vi "WriteHiSpeedDevice.vi"(4 "High Output Pins":T1, 5 "Data Control":T3, 6 "Wait Data Write":T2, 7 "Init Condition":T4 {"Chip Select Pin" items=["ADBUS3 Chip Select", "ADBUS4 GPIOL1", "ADBUS5 GPIOL2", "ADBUS6 GPIOL3", "ADBUS7 GPIOL4"]}, 8 "error in (no error)":errorcluster, 9 "Data Buffer":u8[](array[numeric]), 10 "Control Buffer":u8[](array[numeric]), 11 "Handle":u32) -> (0 "error out":errorcluster, 3 "Result":u32)   [LabVIEW 2010]
uses:
  FTCSPI.dll
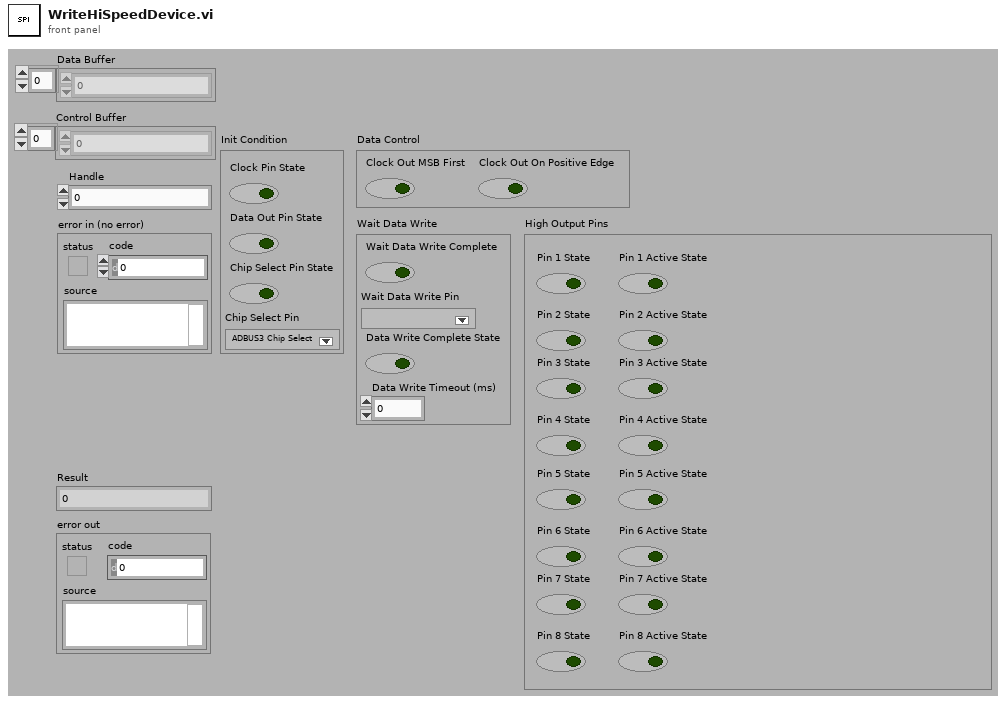
[diagram p1: front panel]
types:
  T1 = cluster{"Pin 1 State":bool, "Pin 1 Active State":bool, "Pin 2 State":bool, "Pin 2 Active State":bool, "Pin 3 State":bool, "Pin 3 Active State":bool, "Pin 4 State":bool, "Pin 4 Active State":bool, "Pin 5 State":bool, "Pin 5 Active State":bool, "Pin 6 State":bool, "Pin 6 Active State":bool, "Pin 7 State":bool, "Pin 7 Active State":bool, "Pin 8 State":bool, "Pin 8 Active State":bool}
  T2 = cluster{"Wait Data Write Complete":bool, "Wait Data Write Pin":u16, "Data Write Complete State":bool, "Data Write Timeout (ms)":u32}
  T3 = cluster{"Clock Out MSB First":bool, "Clock Out On Positive Edge":bool}
  T4 = cluster{"Clock Pin State":bool, "Data Out Pin State":bool, "Chip Select Pin State":bool, "Chip Select Pin":u16}
  T5 = cluster{u32, "Wait Data Write Pin":u16, u32, "Data Write Timeout (ms)":u32}
  T6 = cluster{"[0]":u32, "[1]":u32, "[2]":u32, "[3]":u32, "[4]":u32, "[5]":u32, "[6]":u32, "[7]":u32, "[8]":u32}
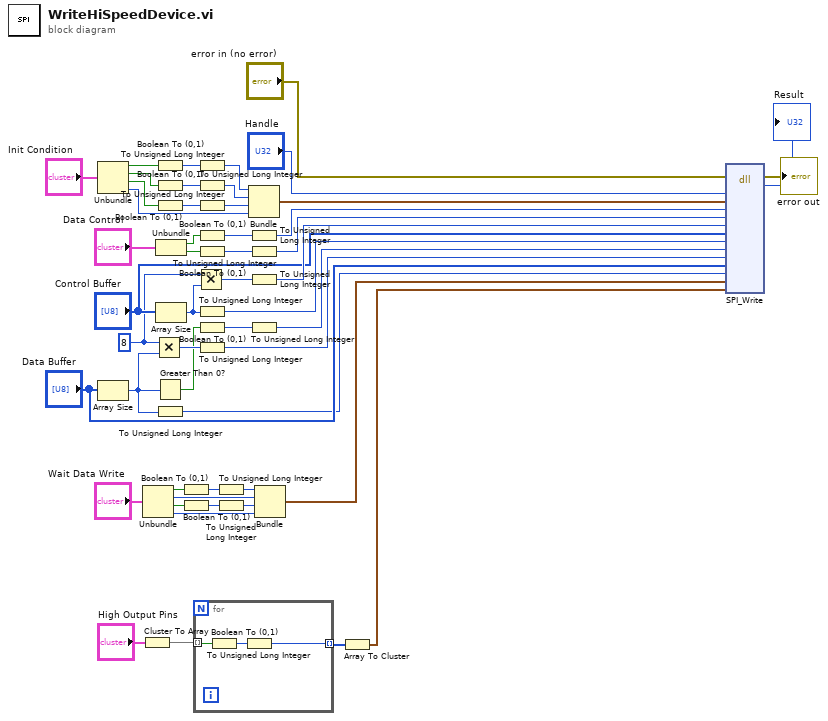
[diagram p0: block diagram]
diagram:
  w23 = 8
  n1 = Unbundle("Init Condition") -> ("Clock Pin State"=w48:bool, "Data Out Pin State"=w47:bool, "Chip Select Pin State"=w46:bool, "Chip Select Pin"=w42:u16)
  n2 = Array Size(array="Data Buffer") -> (size(s)=w17:i32)
  n3 = Cluster To Array(cluster="High Output Pins") -> (array=w5:bool[])
  n4 = Unbundle("Wait Data Write") -> ("Wait Data Write Complete"=w15:bool, "Wait Data Write Pin"=w9:u16, "Data Write Complete State"=w14:bool, "Data Write Timeout (ms)"=w8:u32)
  n5 = Multiply(x=w23, y=w17) -> (x*y=w24:i32)
  n6 = Boolean To (0,1)(Boolean=w48) -> (0, 1=w45:i16)
  n7 = Boolean To (0,1)(Boolean=w47) -> (0, 1=w43:i16)
  n8 = Boolean To (0,1)(Boolean=w46) -> (0, 1=w44:i16)
  n9 = Greater Than 0?(x=w17) -> (x > 0?=w21:bool)
  n10 = To Unsigned Long Integer(number=w17) -> (unsigned 32bit integer=w18:u32)
  n11 = Unbundle("Data Control") -> ("Clock Out MSB First"=w34:bool, "Clock Out On Positive Edge"=w33:bool)
  n12 = Array Size(array="Control Buffer") -> (size(s)=w28:i32)
  n13 = Boolean To (0,1)(Boolean=w15) -> (0, 1=w13:i16)
  n14 = Boolean To (0,1)(Boolean=w14) -> (0, 1=w12:i16)
  n15 = for {
    tunnel: w5 -> [w53] mode=indexing
    tunnel: [w52] -> w4 mode=indexing
    n16 = Boolean To (0,1)(Boolean=w53) -> (0, 1=w54:i16)
    n17 = To Unsigned Long Integer(number=w54) -> (unsigned 32bit integer=w52:u32)
  }
  n18 = Multiply(x=w23, y=w28) -> (x*y=w30:i32)
  n19 = To Unsigned Long Integer(number=w45) -> (unsigned 32bit integer=w39:u32)
  n20 = To Unsigned Long Integer(number=w43) -> (unsigned 32bit integer=w40:u32)
  n21 = To Unsigned Long Integer(number=w44) -> (unsigned 32bit integer=w41:u32)
  n22 = Boolean To (0,1)(Boolean=w34) -> (0, 1=w36:i16)
  n23 = Boolean To (0,1)(Boolean=w33) -> (0, 1=w35:i16)
  n24 = To Unsigned Long Integer(number=w28) -> (unsigned 32bit integer=w27:u32)
  n25 = Boolean To (0,1)(Boolean=w21) -> (0, 1=w20:i16)
  n26 = To Unsigned Long Integer(number=w24) -> (unsigned 32bit integer=w22:u32)
  n27 = To Unsigned Long Integer(number=w13) -> (unsigned 32bit integer=w11:u32)
  n28 = To Unsigned Long Integer(number=w12) -> (unsigned 32bit integer=w10:u32)
  n29 = Bundle(w39, w40, w41, "Chip Select Pin"=w42) -> (w38:cluster{u32, u32, u32, "Chip Select Pin":u16})  [unwired: 1 in]
  n30 = To Unsigned Long Integer(number=w36) -> (unsigned 32bit integer=w32:u32)
  n31 = To Unsigned Long Integer(number=w35) -> (unsigned 32bit integer=w31:u32)
  n32 = To Unsigned Long Integer(number=w30) -> (unsigned 32bit integer=w29:u32)
  n33 = To Unsigned Long Integer(number=w20) -> (unsigned 32bit integer=w19:u32)
  n34 = Bundle(w11, "Wait Data Write Pin"=w9, w10, "Data Write Timeout (ms)"=w8) -> (w7:T5)  [unwired: 1 in]
  n35 = Array To Cluster(array=w4) -> (cluster=w3:T6)
  n36 = dll-call lib="C:/Users/Administrator/Documents/GitHub/labview/FPGA/FTCSPI.dll" fn="SPI_Write"(error in="error in (no error)", "handle"="Handle", "writeStartCondition"=w38, "clockOutDataBitsMSBFirst"=w32, "clockOutDataBitsPosEdge"=w31, "numControlBits"=w29, "controlBuffer"="Control Buffer", "controlBufferSize"=w27, "writeDataBits"=w19, "numDataBits"=w22, "dataBuffer"="Data Buffer", "dataBufferSize"=w18, "waitDataWriteComplete"=w7, "highPinsWriteActiveState"=w3) -> (error out=→"error out":errorcluster, "result"=→"Result":u32)  [unwired: 15 in, 1 out]
